vi "ParseBranchResponse.vi"(5 "body":string, 6 "error in":errorcluster) -> (0 "error out":errorcluster, 4 "branch":T1)   [LabVIEW 2014, in "Raspberry Pi Compatible Compiler for LabVIEW.lvlib" / "GitHub API.lvlib"]
uses:
  GitHub API.lvlib
  TypeDefs/GitHubBranch_TD.ctl
  TypeDefs/GitHubBranchCommit_TD.ctl
  TypeDefs/GitHubCommitCommit_TD.ctl
  TypeDefs/GitHubAuthor_TD.ctl
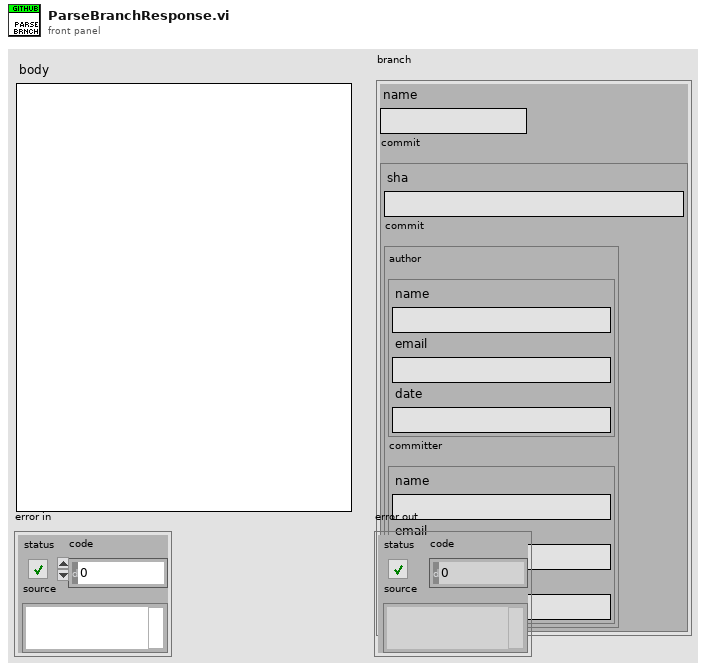
[diagram p1: front panel]
types:
  T1 = typedef "Raspberry Pi Compatible Compiler for LabVIEW.lvlib/GitHub API.lvlib/GitHubBranch_TD.ctl" = cluster{"name":string, "commit":T2}
  T2 = typedef "Raspberry Pi Compatible Compiler for LabVIEW.lvlib/GitHub API.lvlib/GitHubBranchCommit_TD.ctl" = cluster{"sha":string, "commit":T3}
  T3 = typedef "Raspberry Pi Compatible Compiler for LabVIEW.lvlib/GitHub API.lvlib/GitHubCommitCommit_TD.ctl" = cluster{"author":T4, "committer":T4}
  T4 = typedef "Raspberry Pi Compatible Compiler for LabVIEW.lvlib/GitHub API.lvlib/GitHubAuthor_TD.ctl" = cluster{"name":string, "email":string, "date":string}
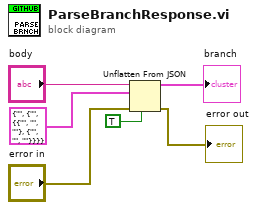
[diagram p0: block diagram]
diagram:
  n1 = Unflatten From JSON(JSON string="body", type and defaults=T1 {"name"="", "commit"={"sha"="", "commit"={"author"={"name"="", "email"="", "date"=""}, "committer"={"name"="", "email"="", "date"=""}}}} ("branch"), default null elements? (F)=TRUE, error in (no error)="error in") -> (value=→"branch":T1, error out=→"error out":errorcluster)  [unwired: 3 in]
